vi "Set Task Timing.vi"(0 "task in":refnum<k21>, 1 "sample mode":i32, 2 "block size":i32, 5 "sample rate":dbl, 11 "error in":errorcluster) -> (4 "task out":refnum<k21>, 6 "actual sample rate":dbl, 15 "error out":errorcluster)   [LabVIEW 2024, in "Dynamic Signal Acquisition (Interactive) UI.lvlib"]
doc: "Set sample rate on task and get actual sample rate."
uses:
  Dynamic Signal Acquisition (Interactive) UI.lvlib
  <resource>/objmgr/daqmx.rc
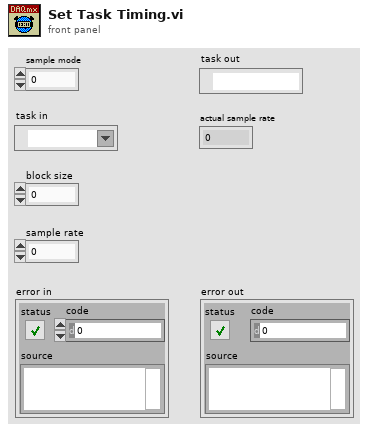
[diagram p1: front panel]
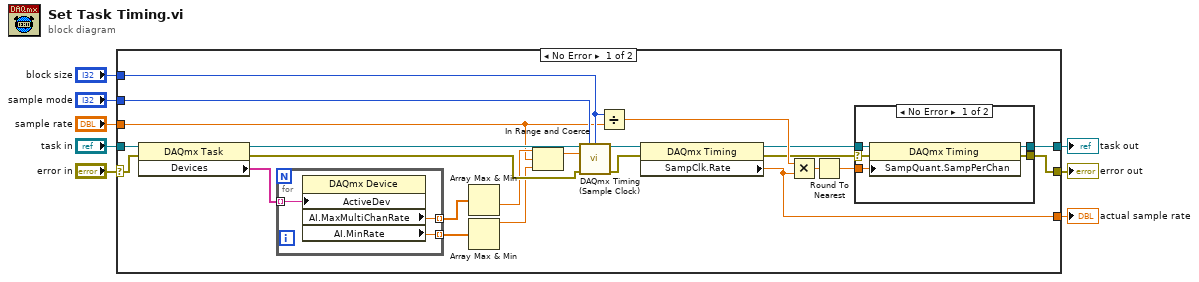
[diagram p0: block diagram]
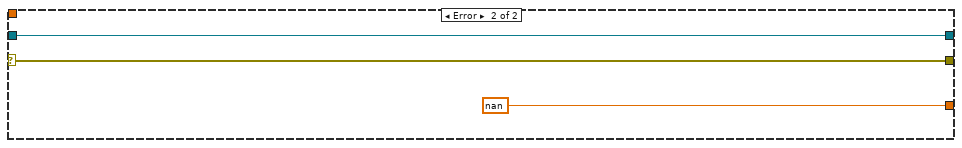
[diagram p3: hidden frame]
diagram:
  n1 = case shown="No Error" "error in" {
    selector: "error in" -> [w24 w43]
    tunnel: "task in" -> [w23 w44]
    tunnel: "sample mode" -> [w19 _]
    tunnel: "block size" -> [w18 _]
    tunnel: "sample rate" -> [w17 _]
    tunnel: [w15 nan ("SampClk.Rate")] -> w3
    tunnel: [w11 w43] -> w2
    tunnel: [w10 w44] -> w1
    frame No Error {
      n2 = property class="DAQmx Task"(reference=w23, error in=w24) -> (reference out=w28:refnum<k21>, error out=w31:errorcluster, "Devices"=w22:tag[])
      n3 = for {
        tunnel: w22 -> [w41] mode=indexing
        tunnel: [w40] -> w25 mode=indexing
        tunnel: [w39] -> w29 mode=indexing
        n4 = property class="DAQmx Device"("ActiveDev"=w41) -> ("AI.MaxMultiChanRate"=w39:dbl, "AI.MinRate"=w40:dbl)  [unwired: 2 in, 2 out]
      }
      n5 = Array Max & Min(array=w29) -> (min value=w30:dbl)  [unwired: 3 out]
      n6 = Array Max & Min(array=w25) -> (max value=w27:dbl)  [unwired: 3 out]
      n7 = In Range and Coerce(upper limit=w30, x=w17, lower limit=w27) -> (coerced(x)=w26:dbl)  [unwired: 1 out]
      n8 = call <vilib>:"DAQmx Timing (Sample Clock).vi"("task/channels in"=w28, "sample mode"=w19, "samples per channel"=w18, "rate"=w26, "error in"=w31) -> ("task out"=w20:refnum<k21>, "error out"=w21:errorcluster)  [unwired: 9 in]
      n9 = Divide(x=w18, y=w17) -> (x/y=w16:dbl)
      n10 = property class="DAQmx Timing"(reference=w20, error in=w21) -> (reference out=w13:refnum<k21>, error out=w12:errorcluster, "SampClk.Rate"=w15:dbl)
      n11 = Multiply(x=w16, y=w15) -> (x*y=w14:dbl)
      n12 = Round To Nearest(number=w14) -> (nearest integer value=w9:dbl)
      n13 = case shown="No Error" w12 {
        selector: w12 -> [w35 w37]
        tunnel: w13 -> [w36 w38]
        tunnel: [w34 w37] -> w11
        tunnel: [w33 w38] -> w10
        tunnel: w9 -> [w32 _]
        frame No Error {
          n14 = property class="DAQmx Timing"(reference=w36, error in=w35, "SampQuant.SampPerChan"=w32) -> (reference out=w33:refnum<k21>, error out=w34:errorcluster)
        }
        frame Error {
        }
      }
    }
    frame Error {
    }
  }
  "task out" <- w1
  "error out" <- w2
  "actual sample rate" <- w3
